vi "Camera Image Acquisition.vi"(10 "Image Size":T4={"H Bin"=1.0, "V Bin"=1.0, "Left"=1.0, "Right"=1024.0, "Top"=1.0, "Bottom"=1024.0} {"V Bin" min=0.0; "H Bin" min=0.0 step=1.0}, 11 "Acquisition Parameters":T5={"Readout Mode"=enum."Image", "Set Acquisition Mode"=enum."Single Scan", "Trigger Mode"=enum."Internal", "Exposure Time (s)"=1.0, "Accumulation Cycle (s)"=1.0, "Kinetic Cycle Time (s)"=1.0, "Number of Kinetics"=1, "Number of Accumulations"=1, "Set VS Speed"=1, "Pixel Rate"=enum."Standard CCD 3 Mhz 14 bits", "V Shift Amplitude"=enum."+1", "Preamp Gain"=enum."1.0"}) -> (0 "Error Out":errorcluster, 1 "File properties":T1, 2 "Image Size 2":T2 {"V Bin" min=0.0; "H Bin" min=0.0 step=1.0}, 3 "Continue with acq?":bool)   [LabVIEW 2014]
uses:
  SubVIs/ctt's/image acquisition 3.ctl
  SubVIs/ctt's/image acquisiton 4.ctl
  SubVIs/ctt's/image acquisition 5.ctl
  SubVIs/ctt's/acquisition control.ctl
  SubVIs/ctt's/image-acquision 2.ctl
  <vilib>/vision/Image Controls.llb/IMAQ Image.ctl
  SubVIs/Initilize Globals.vi
panel:
  in  "High Capacity?":bool
  in  "Shutter":i32(ring) items=["Auto", "Stay Open", "Always Closed"]
  out "Actual Exposure Time (sec)":dbl
  in  "STOP":bool
  in  "Preview":bool
  in  "Go":bool
  in  "Laser Shutter":T3=enum."OFF"
  in  "Number of preview windows":i32=1
  in  "Set to AOI":bool
  in  "Set to 512 x 300":bool
  in  "Set to Maximum":bool
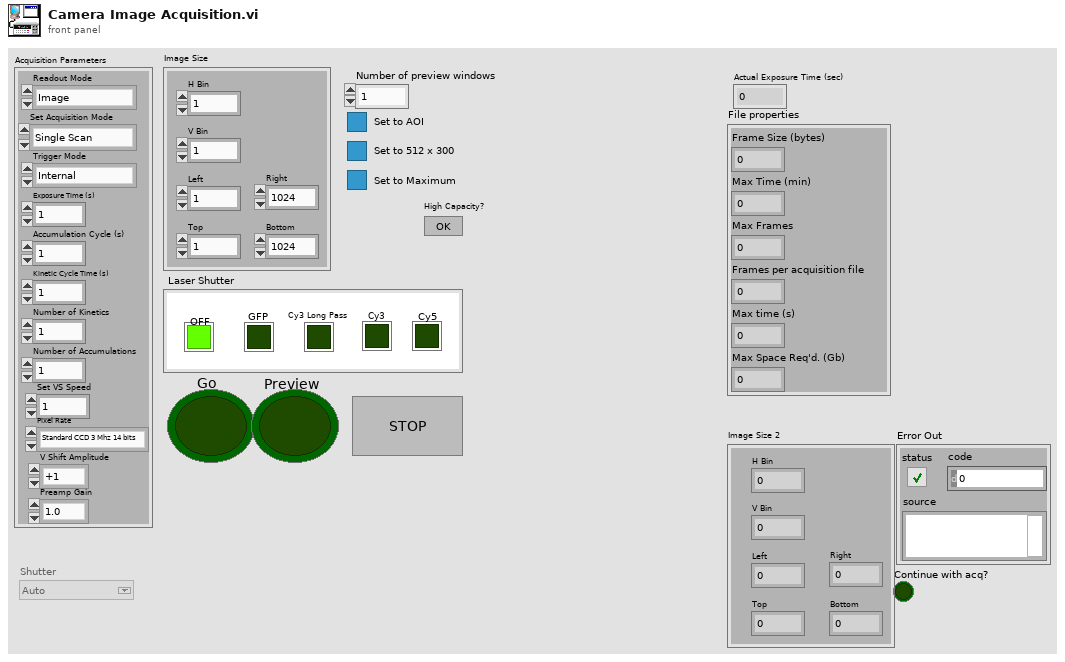
[diagram p1: front panel]
types:
  T1 = cluster{"Frame Size (bytes)":i32, "Max Time (min)":i32, "Max Frames":i32, "Frames per acquisition file":i32, "Max time (s)":i32, "Max Space Req'd. (Gb)":dbl}
  T2 = typedef "acquisition control.ctl" = cluster{"H Bin":dbl, "V Bin":dbl, "Left":dbl, "Right":dbl, "Top":dbl, "Bottom":dbl}
  T3 = typedef "image acquisition 5.ctl" = enum32{"GFP", "Cy3 Long Pass", "Cy3", "Cy5", "OFF"}
  T4 = typedef "image acquisiton 4.ctl" = cluster{"H Bin":dbl, "V Bin":dbl, "Left":dbl, "Right":dbl, "Top":dbl, "Bottom":dbl}
  T5 = typedef "image acquisition 3.ctl" = cluster{"Readout Mode":enum16{"Full Vertical Binning", "Multi-Track", "Random-Track", "Single-Track", "Image"}, "Set Acquisition Mode":enum16{"(do nothing)", "Single Scan", "Accumulate", "Kinetics", "Fast Kinetics", "Run till abort"}, "Trigger Mode":enum16{"Internal", "External"}, "Exposure Time (s)":dbl, "Accumulation Cycle (s)":dbl, "Kinetic Cycle Time (s)":dbl, "Number of Kinetics":i32, "Number of Accumulations":i32, "Set VS Speed":i32, "Pixel Rate":enum16{"EM CCD 10 Mhz 14 bits", "EM CCD 5 Mhz 14 bits", "EM CCD 3 Mhz 14 bits", "EM CCD 1 Mhz 16 bits", "Standard CCD 3 Mhz 14 bits", "Standard CCD 1 Mhz 16 bits"}, "V Shift Amplitude":enum16{"normal", "+1", "+2", "+3", "+4"}, "Preamp Gain":enum16{"1.0", "2.4", "5.0"}}
  T6 = typedef "image-acquision 2.ctl" = u32
  T7 = typedef "IMAQ Image.ctl" = refnum<image>
  T8 = cluster{"H Bin":dbl, "V Bin":dbl, "Left":dbl, "Right":dbl, "Top":dbl, "Bottom":dbl}
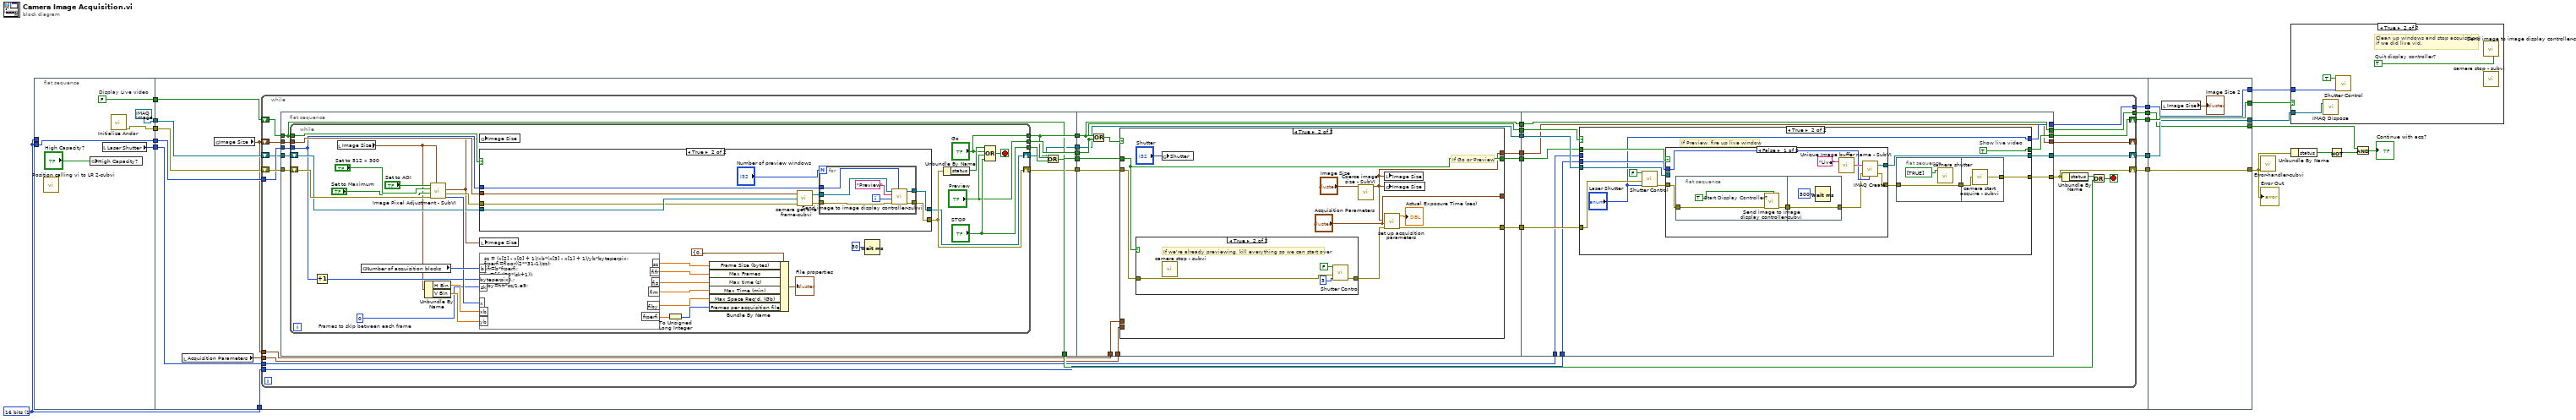
[diagram p0: block diagram]
diagram:
  w1 = T6 1 items=["8 bits", "16 bits", "Float", "Complex", "RGB", "HSL"] ("Image Type")
  n1 = flat-sequence {
    tunnel: [w25] -> w19
    tunnel: [w24] -> w18
    tunnel: w1 -> [w24]
    tunnel: [T7 refnum ("Image")] -> w17
    tunnel: [w23] -> w16
    tunnel: [w21] -> w3
    tunnel: w1 -> [_]
    tunnel: w19 -> [w38]
    tunnel: w18 -> [w37]
    tunnel: w17 -> [w36]
    tunnel: w16 -> [w33]
    tunnel: w1 -> [w34]
    tunnel: [w32] -> w15
    tunnel: [w31] -> w14
    tunnel: [w30] -> w13
    tunnel: [w29] -> w12
    tunnel: [w28] -> w11
    tunnel: w3 -> [w27]
    tunnel: [w212] -> w4
    tunnel: w15 -> [w212]
    tunnel: [w211] -> w2
    tunnel: w14 -> [w211]
    tunnel: [w210] -> w6
    tunnel: w13 -> [w210]
    tunnel: [w209] -> w5
    tunnel: w12 -> [w209]
    tunnel: [w208] -> w10
    tunnel: w11 -> [w208]
    frame #0 {
      w25 = FALSE  # Display Live video
      n2 = call "Position calling vi to LR 2-subvi.vi"() -> ()  [unwired: 4 in, 2 out]
      n3 = global write "Initilize Globals.vi" "High Capacity?"("High Capacity?") -> ()
      n4 = local read "Laser Shutter"() -> (w23:T3)
      n5 = call "Initialize Andor.vi"() -> ("Error Out 2"=w21:errorcluster)  [unwired: 10 in, 1 out]
    }
    frame #1 {
      n6 = local read "Acquisition Parameters"() -> (w35:T5)
      n7 = global read "Initilize Globals.vi" "Image Size"() -> (w26:T8)
      n8 = while {
        shift-right: [w45] -> w31
        shift-left: w27 -> [w67]
        shift-right: [w44] -> w30
        shift-left: w38 -> [w66]
        tunnel: w37 -> [w65]
        shift-right: [w43] -> w29
        shift-left: w36 -> [w64]
        shift-right: [w41] -> _
        shift-left: w26 -> [w63]
        tunnel: w26 -> [w53]
        tunnel: w35 -> [w52]
        tunnel: w34 -> [w47]
        tunnel: w33 -> [w46]
        tunnel: [w42] -> w32
        tunnel: [w39] -> w28
        stop <- w60 stop-if-true
        n9 = flat-sequence {
          tunnel: w67 -> [w78]
          tunnel: w66 -> [w69]
          tunnel: w65 -> [w77]
          tunnel: w64 -> [w76]
          tunnel: w63 -> [w75]
          tunnel: [w73] -> w62
          tunnel: [w72] -> w61
          tunnel: [w71] -> w59
          tunnel: [w70] -> w57
          tunnel: [w69] -> w56
          tunnel: [w68] -> w51
          tunnel: w62 -> [w140]
          tunnel: w61 -> [w141]
          tunnel: w57 -> [w135]
          tunnel: w56 -> [w138]
          tunnel: [w141] -> w55
          tunnel: [w140] -> w54
          tunnel: w53 -> [w137]
          tunnel: w52 -> [w136]
          tunnel: w51 -> [w134]
          tunnel: [w134] -> w50
          tunnel: [w133] -> w49
          tunnel: [w132] -> w48
          tunnel: [w131] -> w40
          tunnel: w55 -> [w170]
          tunnel: w54 -> [w171]
          tunnel: w50 -> [w169]
          tunnel: [w170] -> w39
          tunnel: w49 -> [w168]
          tunnel: w48 -> [w167]
          tunnel: w47 -> [w166]
          tunnel: w46 -> [w165]
          tunnel: [w164] -> w45
          tunnel: [w163] -> w44
          tunnel: [w162] -> w43
          tunnel: [w161] -> w42
          tunnel: [w160] -> w41
          tunnel: w40 -> [w160]
          frame #0 {
            n10 = while {
              shift-right: [w89] -> w70
              shift-left: w78 -> [w111]
              tunnel: w69 -> [w94]
              tunnel: w77 -> [w90]
              shift-right: [w88] -> w68
              shift-left: w76 -> [w93]
              tunnel: w75 -> [w92]
              tunnel: ["STOP"] -> w74
              tunnel: ["Go"] -> w72
              tunnel: ["Preview"] -> w73
              stop <- w86 stop-if-true
              w103 = u16 0  # Frames to skip between each frame
              n11 = Increment(x=w90) -> (x+1=w102:T6)
              n12 = local read "Image Size"() -> (w80:T4)
              n13 = global read "Initilize Globals.vi" "Number of acquisition blocks"() -> (w107:i8)
              n14 = Unbundle By Name(w80) -> ("H Bin"=w105:dbl, "V Bin"=w104:dbl)
              n15 = call "Image Pixel Adjustment - SubVI.vi"("Image Size"=w80, "error in"=w111, "Set to Maximum"="Set to Maximum", "Set to 512 x 300"="Set to 512 x 300", "Set to AOI"="Set to AOI") -> ("Pixels Out"=w106:i32[], "Error Out (no error)"=w91:errorcluster, "Image Size 2"=w79:T8)  [unwired: 4 in]
              n16 = global write "Initilize Globals.vi" "Image Size"(w79) -> ()
              n17 = case shown="True" w94 {
                tunnel: w93 -> [w114 w123]
                tunnel: [w114 w117] -> w88
                tunnel: w92 -> [_ w115]
                tunnel: w91 -> [w113 w122]
                tunnel: w90 -> [_ w118]
                tunnel: [w113 w116] -> w89
                frame False {
                }
                frame True {
                  n18 = call "camera get one frame-subvi.vi"("error in"=w122, "New Image"=w123, "Image Size"=w115) -> ("error out"=w119:errorcluster, "Image Out"=w120:T7)
                  n19 = for {
                    N: "Number of preview windows" -> [_]
                    tunnel: w120 -> [w128]
                    tunnel: w119 -> [w129]
                    tunnel: w118 -> [w130]
                    tunnel: [w125] -> w117
                    tunnel: [w124] -> w116
                    i -> [w126]
                    n20 = call "Send image to image display controller-subvi.vi"("Image"=w128, "Window Title"="Preview" ("Window Title\n(Window only)"), "Window Number"=w126, "error in"=w129, "Image Type"=w130) -> ("Image Out"=w125:T7, "error out"=w124:errorcluster)  [unwired: 4 in]
                  }
                }
              }
              n21 = local write "Image Size"(w79) -> ()
              n22 = formula code="sz = (x[2] - x[0] + 1)/xb*(x[3] - x[1] + 1)/yb*byteperpix;\nfrperfi=floor((2**31-1)/sz);\nfifr=b*frperfi;\nfis=fifr/(30*(sk+1));\nfim=fis/60.;\nfiby=fifr*sz/1.e9;"("x"=w106, "b"=w107, "sk"=w103, "xb"=w105, "yb"=w104, "byteperpix"=w102) -> ("sz"=w95:dbl, "fifr"=w96:dbl, "fis"=w97:dbl, "fim"=w98:dbl, "fiby"=w99:dbl, "frperfi"=w101:dbl)
              n23 = To Unsigned Long Integer(number=w101) -> (unsigned 32bit integer=w100:u32)
              n24 = Bundle By Name(cluster=T1 {"Frame Size (bytes)"=0, "Max Time (min)"=0, "Max Frames"=0, "Frames per acquisition file"=0, "Max time (s)"=0, "Max Space Req'd. (Gb)"=0.0}, "Frame Size (bytes)"=w95, "Max Frames"=w96, "Max time (s)"=w97, "Max Time (min)"=w98, "Max Space Req'd. (Gb)"=w99, "Frames per acquisition file"=w100) -> (→"File properties":T1)
              n25 = Wait (ms)(milliseconds to wait=u32 30) -> ()  [unwired: 1 out]
              n26 = Unbundle By Name(w89) -> ("status"=w87:bool)
              n27 = Compound Arithmetic op=OR(w87, "Go", "Preview", "STOP") -> (w86:bool)
            }
            n28 = Or(x=w72, y=w74) -> (x .or. y?=w71:bool)
          }
          frame #1 {
            n29 = Or(x=w141, y=w140) -> (x .or. y?=w139:bool)
            n30 = case shown="True" w139 {
              tunnel: w138 -> [w145 w154]
              tunnel: [w145 w154] -> w132
              tunnel: [w143 "Acquisition Parameters"] -> _
              tunnel: [w144 w146] -> w131
              tunnel: w137 -> [w144 _]
              tunnel: w136 -> [w143 _]
              tunnel: w135 -> [w142 w150]
              tunnel: [w142 w147] -> w133
              frame False {
              }
              frame True {
                # "If Go or Preview"
                n31 = case shown="True" w154 {
                  tunnel: w150 -> [w155 w159]
                  tunnel: [w155 w157] -> w149
                  frame False {
                  }
                  frame True {
                    # "If we're already previewing, kill everything so we can start over"
                    n32 = call "camera stop - subvi.vi"() -> ()  [unwired: 1 in]
                    n33 = call "Shutter Control.vi"("Laser Shutter"=3, "error in"=w159, "Camera Shutter"=FALSE) -> ("error out"=w157:errorcluster)  [unwired: 8 in]
                  }
                }
                n34 = global write "Initilize Globals.vi" "Shutter"("Shutter") -> ()
                n35 = call "Coerce image size - SubVI.vi"("Image Size"="Image Size") -> ("Image Size 2"=w146:T8)  [unwired: 10 in]
                n36 = local write "Image Size"(w146) -> ()
                n37 = global write "Initilize Globals.vi" "Image Size"(w146) -> ()
                n38 = call "set up acquisition parameters.vi"("error in (no error)"=w149, "Acquisition Parameters"="Acquisition Parameters", "Image Size"=w146) -> ("error out"=w147:errorcluster, "Exposure"=→"Actual Exposure Time (sec)":dbl)  [unwired: 2 in, 3 out]
              }
            }
          }
          frame #2 {
            n39 = case shown="True" w171 {
              tunnel: w169 -> [w172 w183]
              tunnel: w168 -> [w175 w186]
              tunnel: w167 -> [w173 w187]
              tunnel: [w175 w177] -> w164
              tunnel: w166 -> [_ w182]
              tunnel: [w173 w181] -> w163
              tunnel: [w174 "Laser Shutter"] -> w161
              tunnel: w165 -> [w174 _]
              tunnel: [w172 w176] -> w162
              frame False {
              }
              frame True {
                w181 = TRUE  # Show live video
                # "If Preview, fire up live window"
                n40 = call "Shutter Control.vi"("Laser Shutter"="Laser Shutter", "error in"=w186, "Camera Shutter"=FALSE) -> ("error out"=w184:errorcluster)  [unwired: 8 in]
                n41 = case shown="False" w187 {
                  tunnel: w184 -> [w199 w205]
                  tunnel: w183 -> [_ w206]
                  tunnel: [w196 w206] -> w176
                  tunnel: [w197 w205] -> w179
                  tunnel: w182 -> [w193 _]
                  frame False {
                    n42 = flat-sequence {
                      tunnel: w199 -> [w202]
                      tunnel: [w200] -> w198
                      tunnel: [w204] -> w192
                      tunnel: w198 -> [w204]
                      frame #0 {
                        w201 = TRUE  # Start Display Controller?
                        n43 = call "Send image to image display controller-subvi.vi"("error in"=w202, "Start display controller?"=w201) -> ("error out"=w200:errorcluster)  [unwired: 7 in, 1 out]
                      }
                      frame #1 {
                        n44 = Wait (ms)(milliseconds to wait=u32 500) -> ()  [unwired: 1 out]
                      }
                    }
                    n45 = call "Unique Image buffer name - SubVI.vi"("Buffer  base name"="Live") -> ("Image Name"=w195:string)  [unwired: 1 in]
                    n46 = call "IMAQ Create"("Image Name"=w195, "Image Type"=w193, "error in (no error)"=w192) -> ("New Image"=w196:T7, "error out"=w197:errorcluster)  [unwired: 1 in, 1 out]
                  }
                  frame True {
                  }
                }
                n47 = flat-sequence {
                  tunnel: w179 -> [w189]
                  tunnel: [w189] -> w178
                  tunnel: w178 -> [w191]
                  tunnel: [w190] -> w177
                  frame #0 {
                    n48 = call "camera shutter.vi"("Array"=bool[] [TRUE]) -> ()  [unwired: 10 in, 1 out]
                  }
                  frame #1 {
                    n49 = call "camera start acquire - subvi.vi"("error in"=w191) -> ("error out"=w190:errorcluster)
                  }
                }
              }
            }
          }
        }
        n50 = Unbundle By Name(w45) -> ("status"=w58:bool)
        n51 = Or(x=w58, y=w59) -> (x .or. y?=w60:bool)
      }
    }
    frame #2 {
      n52 = local read "Image Size"() -> (→"Image Size 2":T4)
    }
  }
  n53 = call "Error-handler-subvi.vi"("error in"=w2) -> ()  [unwired: 4 in, 3 out]
  n54 = case shown="True" w6 {
    tunnel: w5 -> [_ w215]
    tunnel: w4 -> [_ w214]
    frame False {
    }
    frame True {
      w216 = TRUE  # Quit display controller?
      # "Clean up windows and stop acquisition\nif we did live vid."
      n55 = call "IMAQ Dispose"("Image"=w215) -> ()  [unwired: 2 in, 4 out]
      n56 = call "Shutter Control.vi"("Laser Shutter"=w214, "Camera Shutter"=TRUE) -> ()  [unwired: 9 in, 1 out]
      n57 = call "Send image to image display controller-subvi.vi"("Quit display controller?"=w216) -> ()  [unwired: 8 in, 2 out]
      n58 = call "camera stop - subvi.vi"() -> ()  [unwired: 1 in]
    }
  }
  n59 = Unbundle By Name(w2) -> ("status"=w9:bool)
  n60 = Not(x=w9) -> (.not. x?=w8:bool)
  n61 = And(x=w10, y=w8) -> (x .and. y?=→"Continue with acq?":bool)
  "Error Out" <- w2
